vi "GaugesTest.vi"() -> ()   [LabVIEW 2019]
uses:
  <vilib>/Instr/_visa.llb/VISA Configure Serial Port (Instr).vi
panel:
  out "Waveform Chart":cluster{dbl, dbl, dbl}(graph)
  in  "termination char\n(0xA = '\\n' = LF)":u8=13 format="%.0x"
  in  "stop bits (10: 1 bit)":u16=10
  in  "flow control (0:none)":dbl
  in  "parity (0:none)":dbl
  in  "data bits (8)":u16=8 min=5 max=8 step=1
  in  "baud rate (9600)":u32=9600
  in  "VISA resource name":refnum<visa-resource-name>
  out "Response G3":string
  out "bytes read 3":u32
  out "Response G2":string
  out "bytes read 2":u32
  in  "Recieve Data":bool
  out "Response G1":string
  out "bytes read":u32
  in  "Stop Program":bool
  # "Values"
  # "Para activar/desactivar la visualización de una gráfica:\nDar click en el ícono que está al lado del nombre de la gráfica y después click en \"Plot Visible\""
  # "Para reiniciar la gráfica: \n-click derecho sobre ella\n-en \"Data Operation\", dar click en \"Clear Chart\""
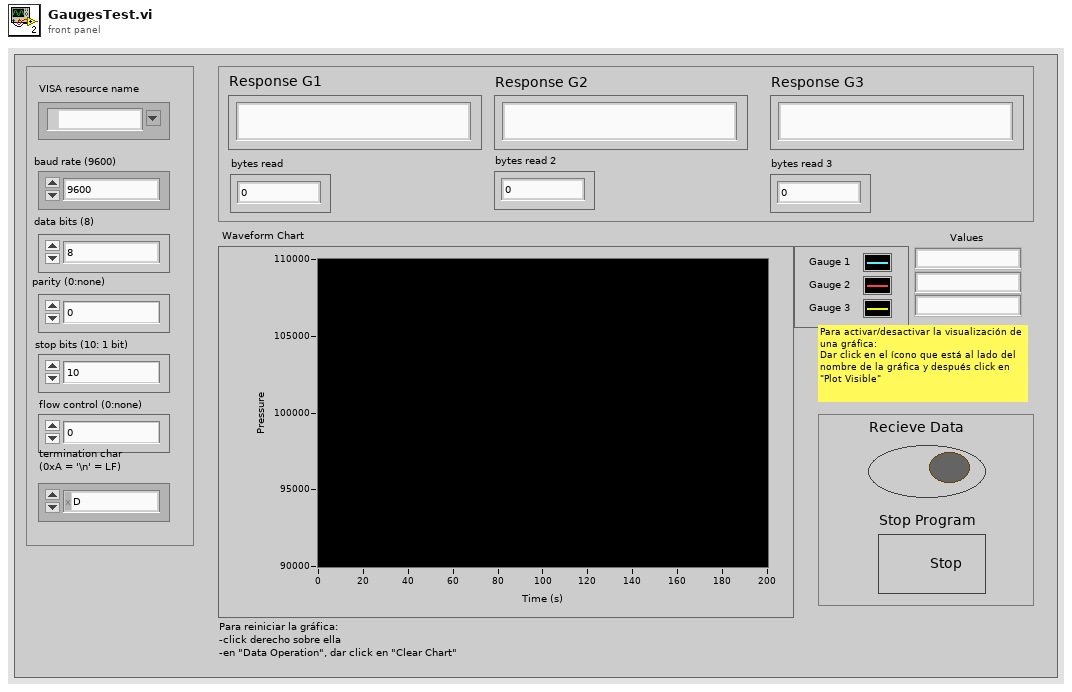
[diagram p1: front panel]
types:
  T1 = enum16{"open", "replace", "create", "open or create", "replace or create", "replace or create with confirmation"}
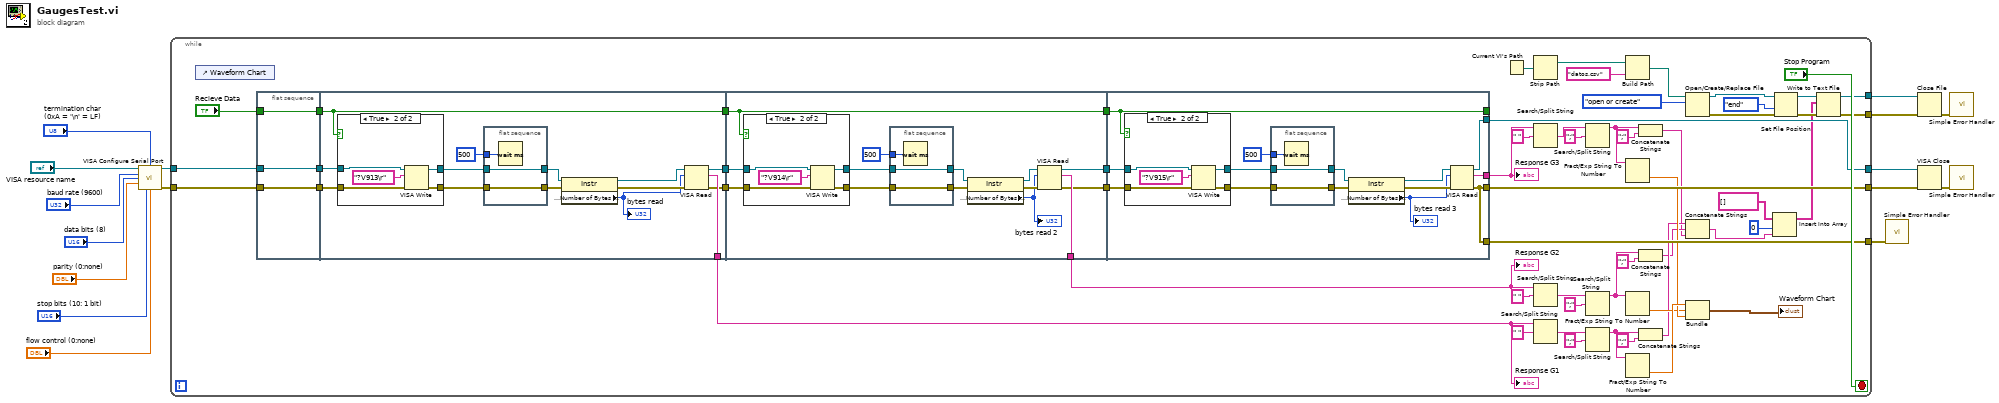
[diagram p0: block diagram]
diagram:
  n1 = call-poly "VISA Configure Serial Port"("VISA resource name"="VISA resource name", "termination char\n(0xA = '\\n' = LF)"="termination char\n(0xA = '\\n' = LF)", "baud rate (9600)"="baud rate (9600)", "data bits (8)"="data bits (8)", "parity (0:none)"="parity (0:none)", "stop bits (10: 1 bit)"="stop bits (10: 1 bit)", "flow control (0:none)"="flow control (0:none)") -> ("VISA resource name out"=w14:refnum<visa-resource-name>, "error out"=w15:errorcluster)  [unwired: 3 in, 4 out]
  n2 = while {
    tunnel: w15 -> [w70]
    tunnel: w14 -> [w69]
    tunnel: [w58] -> w13
    tunnel: [w57] -> w12
    tunnel: [w53] -> w11
    tunnel: [w28] -> w3
    tunnel: [w35] -> w2
    stop <- "Stop Program" stop-if-true
    n3 = control-ref of="Waveform Chart"() -> ()  [unwired: 1 out]
    n4 = flat-sequence {
      tunnel: w69 -> [w74]
      tunnel: w70 -> [w75]
      tunnel: "Recieve Data" -> [w76]
      tunnel: [w76] -> w26
      tunnel: [w75] -> w25
      tunnel: [w74] -> w24
      tunnel: [w80] -> w68
      tunnel: [w79] -> w66
      tunnel: [w78] -> w65
      tunnel: [w77] -> w51
      tunnel: w26 -> [w77]
      tunnel: w25 -> [w85]
      tunnel: w24 -> [w84]
      tunnel: w66 -> [w109]
      tunnel: w65 -> [w108]
      tunnel: [w104] -> w61
      tunnel: [w102] -> w60
      tunnel: [w103] -> w59
      tunnel: w51 -> [w101]
      tunnel: [w101] -> w50
      tunnel: w60 -> [w135]
      tunnel: w59 -> [w134]
      tunnel: [w126] -> w58
      tunnel: [w128] -> w57
      tunnel: [w127] -> w52
      tunnel: [w126] -> w53
      tunnel: w50 -> [w125]
      tunnel: [w125] -> _
      frame #0 {
      }
      frame #1 {
        n5 = case shown="True" w77 {
          tunnel: w85 -> [w91 w97]
          tunnel: w84 -> [w92 w96]
          tunnel: [w91 w95] -> w83
          tunnel: [w92 w93] -> w82
          frame False {
          }
          frame True {
            n6 = VISA Write(VISA resource name=w96, write buffer="?V913\r" ("Command"), error in (no error)=w97) -> (VISA resource name out=w93:refnum<visa-resource-name>, error out=w95:errorcluster)  [unwired: 1 out]
          }
        }
        n7 = flat-sequence {
          tunnel: w83 -> [w99]
          tunnel: [w99] -> w90
          tunnel: u32 500 ("delay before read (ms)") -> [w100]
          tunnel: w82 -> [w98]
          tunnel: [w98] -> w81
          frame #0 {
            n8 = Wait (ms)(milliseconds to wait=w100) -> ()  [unwired: 1 out]
          }
        }
        n9 = property class="Instr"(reference=w81, error in=w90) -> (reference out=w88:refnum<visa-resource-name>, error out=w87:errorcluster, "Serial Settings:Number of Bytes at Serial Port"=w86:u32)
        "bytes read" <- w86
        n10 = VISA Read(VISA resource name=w88, byte count=w86, error in (no error)=w87) -> (VISA resource name out=w79:refnum<visa-resource-name>, read buffer=w80:string, error out=w78:errorcluster)  [unwired: 1 out]
      }
      frame #2 {
        n11 = case shown="True" w101 {
          tunnel: w109 -> [w116 w120]
          tunnel: w108 -> [w115 w119]
          tunnel: [w116 w118] -> w107
          tunnel: [w115 w117] -> w106
          frame False {
          }
          frame True {
            n12 = VISA Write(VISA resource name=w120, write buffer="?V914\r" ("Command"), error in (no error)=w119) -> (VISA resource name out=w118:refnum<visa-resource-name>, error out=w117:errorcluster)  [unwired: 1 out]
          }
        }
        n13 = flat-sequence {
          tunnel: w106 -> [w123]
          tunnel: [w123] -> w105
          tunnel: u32 500 ("delay before read (ms)") -> [w124]
          tunnel: w107 -> [w122]
          tunnel: [w122] -> w111
          frame #0 {
            n14 = Wait (ms)(milliseconds to wait=w124) -> ()  [unwired: 1 out]
          }
        }
        n15 = property class="Instr"(reference=w111, error in=w105) -> (reference out=w114:refnum<visa-resource-name>, error out=w113:errorcluster, "Serial Settings:Number of Bytes at Serial Port"=w112:u32)
        "bytes read 2" <- w112
        n16 = VISA Read(VISA resource name=w114, byte count=w112, error in (no error)=w113) -> (VISA resource name out=w103:refnum<visa-resource-name>, read buffer=w104:string, error out=w102:errorcluster)  [unwired: 1 out]
      }
      frame #3 {
        n17 = case shown="True" w125 {
          tunnel: w135 -> [w139 w144]
          tunnel: w134 -> [w140 w143]
          tunnel: [w139 w142] -> w132
          tunnel: [w140 w141] -> w131
          frame False {
          }
          frame True {
            n18 = VISA Write(VISA resource name=w143, write buffer="?V915\r" ("Command"), error in (no error)=w144) -> (VISA resource name out=w141:refnum<visa-resource-name>, error out=w142:errorcluster)  [unwired: 1 out]
          }
        }
        n19 = flat-sequence {
          tunnel: u32 500 ("delay before read (ms)") -> [w148]
          tunnel: w132 -> [w147]
          tunnel: w131 -> [w146]
          tunnel: [w147] -> w130
          tunnel: [w146] -> w129
          frame #0 {
            n20 = Wait (ms)(milliseconds to wait=w148) -> ()  [unwired: 1 out]
          }
        }
        n21 = property class="Instr"(reference=w129, error in=w130) -> (reference out=w138:refnum<visa-resource-name>, error out=w137:errorcluster, "Serial Settings:Number of Bytes at Serial Port"=w136:u32)
        "bytes read 3" <- w136
        n22 = VISA Read(VISA resource name=w138, byte count=w136, error in (no error)=w137) -> (VISA resource name out=w128:refnum<visa-resource-name>, read buffer=w127:string, error out=w126:errorcluster)  [unwired: 1 out]
      }
    }
    n23 = Current VI's Path() -> (path=w48:path)
    n24 = Strip Path(path=w48) -> (stripped path=w47:path)  [unwired: 1 out]
    n25 = Search/Split String(string=w52, search string/char (-)=" ") -> (match + rest of string=w54:string)  [unwired: 1 in, 2 out]
    n26 = Search/Split String(string=w61, search string/char (-)=" ") -> (match + rest of string=w62:string)  [unwired: 1 in, 2 out]
    n27 = Search/Split String(string=w68, search string/char (-)=" ") -> (match + rest of string=w67:string)  [unwired: 1 in, 2 out]
    n28 = Search/Split String(string=w54, search string/char (-)=";") -> (substring before match=w29:string)  [unwired: 1 in, 2 out]
    n29 = Search/Split String(string=w62, search string/char (-)=";") -> (substring before match=w31:string)  [unwired: 1 in, 2 out]
    n30 = Search/Split String(string=w67, search string/char (-)=";") -> (substring before match=w30:string)  [unwired: 1 in, 2 out]
    n31 = Build Path(base path=w47, name or relative path="datos.csv") -> (appended path=w46:path)
    n32 = Fract/Exp String To Number(string=w29) -> (number=w37:dbl)  [unwired: 3 in, 1 out]
    n33 = Fract/Exp String To Number(string=w31) -> (number=w36:dbl)  [unwired: 3 in, 1 out]
    n34 = Fract/Exp String To Number(string=w30) -> (number=w38:dbl)  [unwired: 3 in, 1 out]
    n35 = Concatenate Strings(w29, ";" ("string")) -> (w18:string)
    n36 = Concatenate Strings(w31, ";" ("string")) -> (w19:string)
    n37 = Concatenate Strings(w30, ";" ("string")) -> (w20:string)
    n38 = Open/Create/Replace File(file path (use dialog)=w46, operation (0:open)=T1."open or create") -> (refnum out=w44:refnum<file>, error out=w42:errorcluster)  [unwired: 4 in, 1 out]
    n39 = Concatenate Strings(w20, w19, w18) -> (w17:string)
    n40 = Bundle(w38, w36, w37) -> (→"Waveform Chart":cluster{dbl, dbl, dbl})  [unwired: 1 in]
    n41 = Insert Into Array(array=string[] [], index=0, new element=w17) -> (w21:string[])
    n42 = Set File Position(refnum=w44, from (0:start)=enum16{"start", "end", "current"}."end", error in=w42) -> (refnum out=w27:refnum<file>, error out=w41:errorcluster)  [unwired: 1 in]
    n43 = Write to Text File(file (use dialog)=w27, text=w21, error in=w41) -> (refnum out=w28:refnum<file>, error out=w35:errorcluster)  [unwired: 1 in, 1 out]
    "Response G1" <- w68
    "Response G2" <- w61
    "Response G3" <- w52
  }
  n44 = call <vilib>:"Simple Error Handler.vi"("error in (no error)"=w11) -> ()  [unwired: 1 in, 8 out]
  n45 = Close File(refnum=w3, error in=w2) -> (error out=w1:errorcluster)  [unwired: 1 out]
  n46 = VISA Close(VISA resource name=w12, error in (no error)=w13) -> (error out=w16:errorcluster)
  n47 = call <vilib>:"Simple Error Handler.vi"("error in (no error)"=w1) -> ()  [unwired: 1 in, 8 out]
  n48 = call <vilib>:"Simple Error Handler.vi"("error in (no error)"=w16) -> ()  [unwired: 1 in, 8 out]
